vi "angleDetection.vi"(5 "error in":errorcluster, 7 "Range (Threshold 1)":cluster{"Lower value":sgl, "Upper value":sgl}={"Lower value"=0.0, "Upper value"=108.0}, 8 "Image In":T1) -> (0 "error out":errorcluster, 1 "Caliper Results (Caliper 2)":sgl[][](array[numeric]) format="%.2f", 2 "Calibrated Results (Caliper 2)":sgl[][](array[numeric]) format="%.2f", 3 "Image Out":T1)   [LabVIEW 2015]
uses:
  <vilib>/vision/Image Controls.llb/IMAQ Image.ctl
  <vilib>/vision/NI_Vision_Development_Module.lvlib
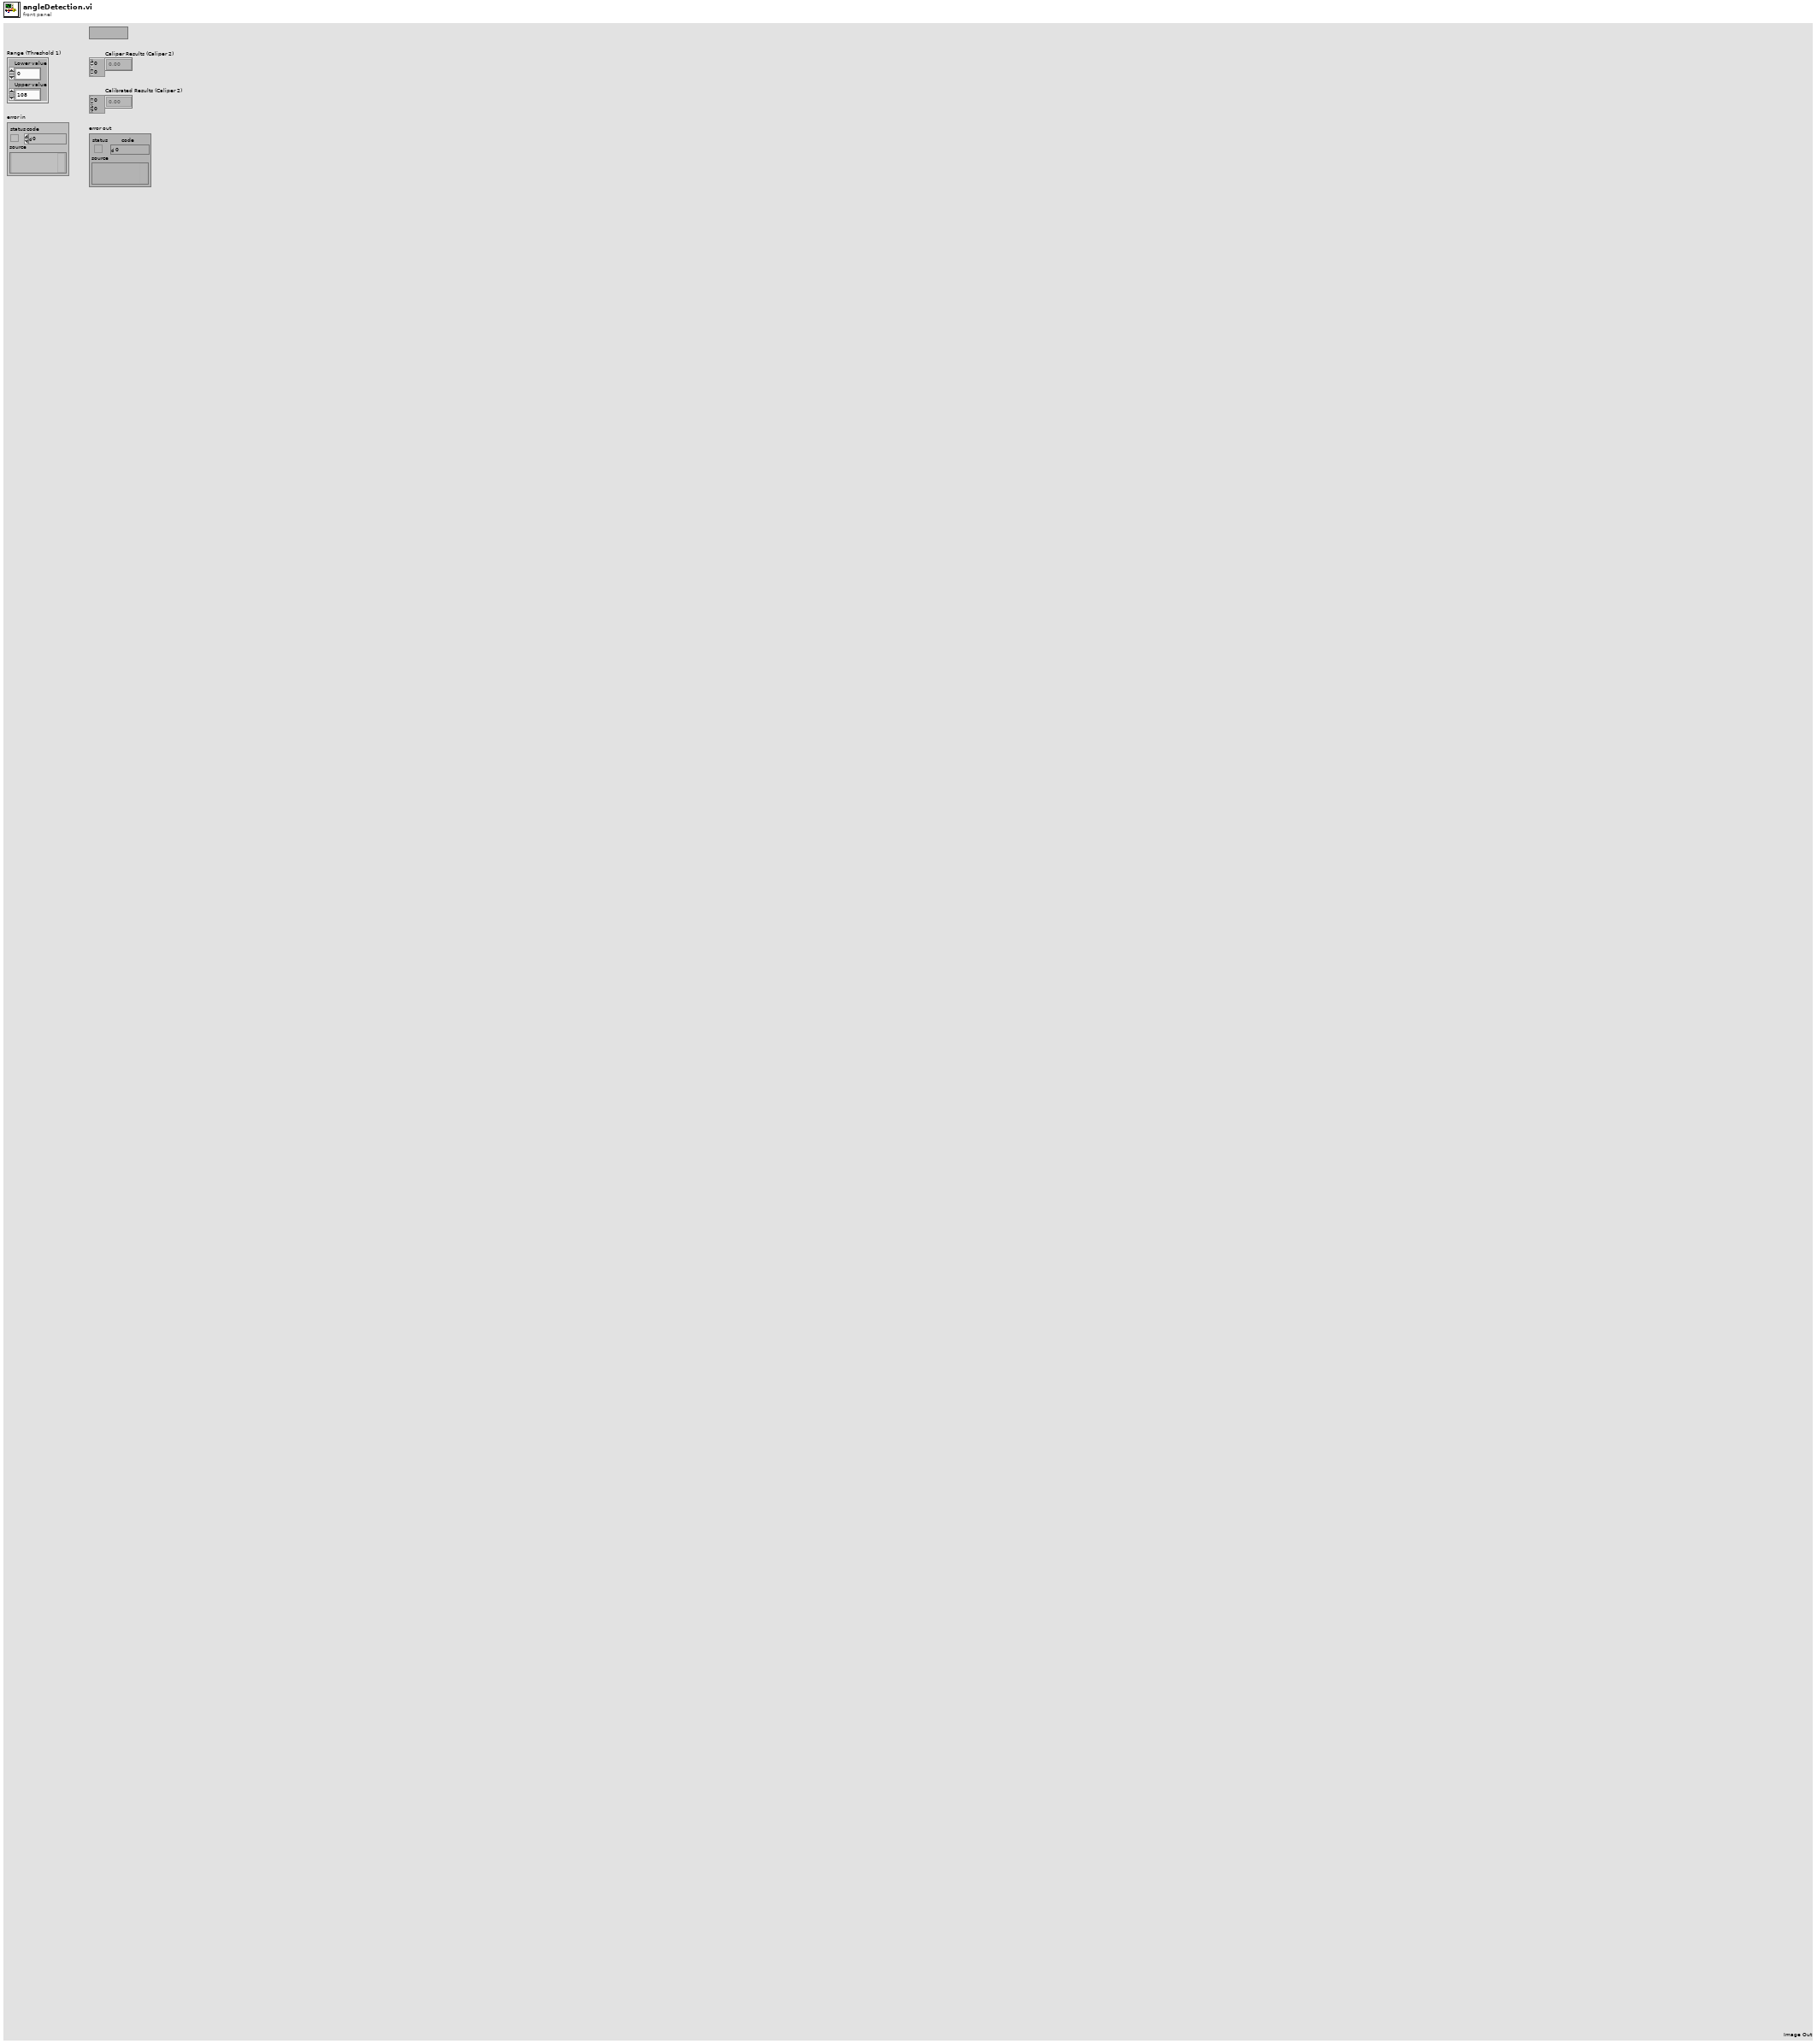
[diagram p1: front panel]
types:
  T1 = typedef "IMAQ Image.ctl" = refnum<image>
  T2 = cluster{"Feature":u32, "Points IDs":cluster{"GUID":string, "Index":i32}[]}[]
  T3 = cluster{"Edge Polarity":u32, "Kernel Size":u32, "Width":u32, "Minimum Edge Strength":sgl, "Interpolation Type":enum32{"Zero Order", "Bilinear", "Quadratic", "Cubic", "Bilinear Fixed"}, "Data Processing Method":enum32{"Average", "Median"}}
  T4 = enum16{"Get First Edge", "Get First + Last Edge", "Get All Edges", "Get Best Edge"}
  T5 = cluster{"Global Rectangle":i32[], "Contours":cluster{"ID":enum32{"External", "Internal"}, "Type":u32, "Coordinates":i32[]}[]}
  T6 = cluster{"Sigma":sgl, "HThresh":sgl, "LThres":sgl, "WindowSize":i32}
  T7 = cluster{"Brightness":sgl, "Contrast":sgl, "Gamma":sgl}
  T8 = typedef "Edge New.ctl" = cluster{"Location (Pixel)":cluster{"X":sgl, "Y":sgl}, "Location (Real-World)":cluster{"X":sgl, "Y":sgl}, "Distance (Pixel)":dbl, "Distance (Real-World)":dbl, "Strength":dbl, "Noise":dbl, "Rising?":bool}
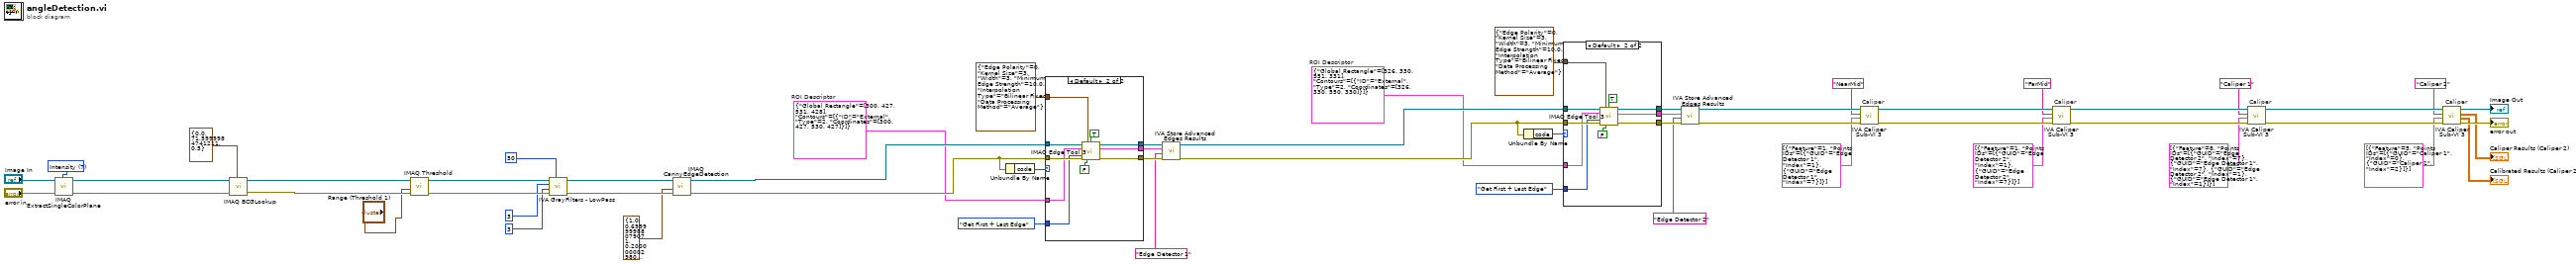
[diagram p0: block diagram]
diagram:
  w21 = T5 {"Global Rectangle"=[326, 330, 551, 331], "Contours"=[{"ID"=enum."External", "Type"=2, "Coordinates"=[326, 330, 550, 330]}]}  # ROI Descriptor
  w31 = T5 {"Global Rectangle"=[300, 427, 531, 428], "Contours"=[{"ID"=enum."External", "Type"=2, "Coordinates"=[300, 427, 530, 427]}]}  # ROI Descriptor
  w57 = 7 items=["Red", "Green", "Blue", "Hue", "Saturation", "Luminance", "Value", "Intensity"] ("Color Plane")
  # "Caliper"
  # "Caliper"
  # "Caliper"
  # "Caliper"
  n1 = call "IMAQ ExtractSingleColorPlane"("Color Plane"=w57, "error in (no error)"="error in", "Image Src"="Image In") -> ("error out"=w54:errorcluster, "Image Dst Out"=w52:T1)  [unwired: 1 in, 6 out]
  n2 = call "IMAQ BCGLookup"("Image Src"=w52, "BCG Values"=T7 {"Brightness"=0.0, "Contrast"=71.6, "Gamma"=0.5}, "error in (no error)"=w54) -> ("Image Dst Out"=w49:T1, "error out"=w53:errorcluster)  [unwired: 2 in, 2 out]
  n3 = call "IMAQ Threshold"("error in (no error)"=w53, "Range"="Range (Threshold 1)", "Image Src"=w49) -> ("error out"=w48:errorcluster, "Image Dst Out"=w47:T1)  [unwired: 3 in, 4 out]
  n4 = call <vilib>:"IVA GrayFilters - LowPass.vi"("Tolerance"=50, "error in"=w48, "Filter size Y"=3, "Filter size X"=3, "Image In"=w47) -> ("error out"=w46:errorcluster, "Image Out"=w42:T1)  [unwired: 5 out]
  n5 = call "IMAQ CannyEdgeDetection"("Image Src"=w42, "Filter Parameters"=T6 {"Sigma"=1.0, "HThresh"=0.7, "LThres"=0.2, "WindowSize"=9}, "error in (no error)"=w46) -> ("Image Dst Out"=w39:T1, "error out"=w41:errorcluster)  [unwired: 1 in, 4 out]
  n6 = Unbundle By Name(w41) -> ("code"=w30:i32)
  n7 = case shown="Default" w30 {
    tunnel: w41 -> [_ w68]
    tunnel: w39 -> [w58 w67]
    tunnel: T4."Get First + Last Edge" ("Process") -> [_ w66]
    tunnel: T3 {"Edge Polarity"=0, "Kernel Size"=3, "Width"=3, "Minimum Edge Strength"=10.0, "Interpolation Type"=enum."Bilinear Fixed", "Data Processing Method"=enum."Average"} ("Edge Options") -> [_ w65]
    tunnel: [_ w64] -> w36
    tunnel: [w58 w63] -> w34
    tunnel: [_ w62] -> w33
    tunnel: w31 -> [_ w61]
    frame -1074396199, -1074396198 {
    }
    frame Default {
      n8 = call "IMAQ Edge Tool 3"("Image"=w67, "Edge Options"=w65, "Optimized Mode"=TRUE, "ROI Descriptor"=w61, "Process"=w66, "error in (no error)"=w68, "Reverse Direction"=FALSE) -> ("Image (duplicate)"=w63:T1, "Edge Information"=w62:T8[], "error out"=w64:errorcluster)  [unwired: 6 out]
    }
  }
  n9 = call <vilib>:"IVA Store Advanced Edges Results.vi"("error in (no error)"=w36, "Step Name"="Edge Detector 1", "Edge Information"=w33, "Image in"=w34) -> ("error out"=w35:errorcluster, "Image dup"=w29:T1)  [unwired: 6 out]
  n10 = Unbundle By Name(w35) -> ("code"=w20:i32)
  n11 = case shown="Default" w20 {
    tunnel: w35 -> [_ w79]
    tunnel: w29 -> [w69 w78]
    tunnel: T4."Get First + Last Edge" ("Process") -> [_ w77]
    tunnel: T3 {"Edge Polarity"=0, "Kernel Size"=3, "Width"=3, "Minimum Edge Strength"=10.0, "Interpolation Type"=enum."Bilinear Fixed", "Data Processing Method"=enum."Average"} ("Edge Options") -> [_ w76]
    tunnel: [_ w75] -> w26
    tunnel: [w69 w74] -> w24
    tunnel: [_ w73] -> w23
    tunnel: w21 -> [_ w72]
    frame -1074396199, -1074396198 {
    }
    frame Default {
      n12 = call "IMAQ Edge Tool 3"("Image"=w78, "Edge Options"=w76, "Optimized Mode"=TRUE, "ROI Descriptor"=w72, "Process"=w77, "error in (no error)"=w79, "Reverse Direction"=FALSE) -> ("Image (duplicate)"=w74:T1, "Edge Information"=w73:T8[], "error out"=w75:errorcluster)  [unwired: 6 out]
    }
  }
  n13 = call <vilib>:"IVA Store Advanced Edges Results.vi"("error in (no error)"=w26, "Step Name"="Edge Detector 2", "Edge Information"=w23, "Image in"=w24) -> ("error out"=w25:errorcluster, "Image dup"=w19:T1)  [unwired: 6 out]
  n14 = call <vilib>:"IVA Caliper Sub-VI 3.vi"("error in"=w25, "Parameters"=T2 [{"Feature"=1, "Points IDs"=[{"GUID"="Edge Detector 1", "Index"=1}, {"GUID"="Edge Detector 1", "Index"=7}]}], "Step Name"="NearMid", "Image In"=w19) -> ("error out"=w18:errorcluster, "Image Out"=w15:T1)  [unwired: 1 in, 5 out]
  n15 = call <vilib>:"IVA Caliper Sub-VI 3.vi"("error in"=w18, "Parameters"=T2 [{"Feature"=1, "Points IDs"=[{"GUID"="Edge Detector 2", "Index"=1}, {"GUID"="Edge Detector 2", "Index"=7}]}], "Step Name"="FarMid", "Image In"=w15) -> ("error out"=w14:errorcluster, "Image Out"=w11:T1)  [unwired: 1 in, 5 out]
  n16 = call <vilib>:"IVA Caliper Sub-VI 3.vi"("error in"=w14, "Parameters"=T2 [{"Feature"=8, "Points IDs"=[{"GUID"="Edge Detector 2", "Index"=7}, {"GUID"="Edge Detector 1", "Index"=7}, {"GUID"="Edge Detector 2", "Index"=1}, {"GUID"="Edge Detector 1", "Index"=1}]}], "Step Name"="Caliper 1", "Image In"=w11) -> ("error out"=w10:errorcluster, "Image Out"=w7:T1)  [unwired: 1 in, 5 out]
  n17 = call <vilib>:"IVA Caliper Sub-VI 3.vi"("error in"=w10, "Parameters"=T2 [{"Feature"=5, "Points IDs"=[{"GUID"="Caliper 1", "Index"=0}, {"GUID"="Caliper 1", "Index"=2}]}], "Step Name"="Caliper 2", "Image In"=w7) -> ("error out"=→"error out":errorcluster, "Results (Calibrated)"=→"Calibrated Results (Caliper 2)":sgl[][], "Results (Pixels)"=→"Caliper Results (Caliper 2)":sgl[][], "Image Out"=→"Image Out":T1)  [unwired: 1 in, 3 out]
